vi "Calibration Read Dates.vi"(0 "Equipment Description":T3, 1 "File Path":path=path "C:/GE/Washer DOE/CalibrationDates.txt", 2 "Manufacturer":T3, 3 "Model Number":T3, 5 "error in (no error)":errorcluster, 8 "Calibration ID":T3, 9 "Serial Number":T2, 10 "Last Calibrated":T1 {"Eq20" format="%<%x>T"; "Eq19" format="%<%x>T"; "Eq18" format="%<%x>T"; "Eq17" format="%<%x>T"; "Eq16" format="%<%x>T"; "Eq15" format="%<%x>T"; "Eq14" format="%<%x>T"; "Eq13" format="%<%x>T"; "Eq12" format="%<%x>T"; "Eq11" format="%<%x>T"; "Eq10" format="%<%x>T"; "Eq9" format="%<%x>T"; "Eq8" format="%<%x>T"; "Eq7" format="%<%x>T"; "Eq6" format="%<%x>T"; "Eq5" format="%<%x>T"; "Eq4" format="%<%x>T"; "Eq3" format="%<%x>T"; "Eq2" format="%<%x>T"; "Eq1" format="%<%x>T"}, 11 "Calibration Due":T1 {"Eq20" format="%<%x>T"; "Eq19" format="%<%x>T"; "Eq18" format="%<%x>T"; "Eq17" format="%<%x>T"; "Eq16" format="%<%x>T"; "Eq15" format="%<%x>T"; "Eq14" format="%<%x>T"; "Eq13" format="%<%x>T"; "Eq12" format="%<%x>T"; "Eq11" format="%<%x>T"; "Eq10" format="%<%x>T"; "Eq9" format="%<%x>T"; "Eq8" format="%<%x>T"; "Eq7" format="%<%x>T"; "Eq6" format="%<%x>T"; "Eq5" format="%<%x>T"; "Eq4" format="%<%x>T"; "Eq3" format="%<%x>T"; "Eq2" format="%<%x>T"; "Eq1" format="%<%x>T"}) -> (14 "output cluster":T4 {"Calibration Due"."Eq20" format="%<%x>T"; "Calibration Due"."Eq19" format="%<%x>T"; "Calibration Due"."Eq18" format="%<%x>T"; "Calibration Due"."Eq17" format="%<%x>T"; "Calibration Due"."Eq16" format="%<%x>T"; "Calibration Due"."Eq15" format="%<%x>T"; "Calibration Due"."Eq14" format="%<%x>T"; "Calibration Due"."Eq13" format="%<%x>T"; "Calibration Due"."Eq12" format="%<%x>T"; "Calibration Due"."Eq11" format="%<%x>T"; "Calibration Due"."Eq10" format="%<%x>T"; "Calibration Due"."Eq9" format="%<%x>T"; "Calibration Due"."Eq8" format="%<%x>T"; "Calibration Due"."Eq7" format="%<%x>T"; "Calibration Due"."Eq6" format="%<%x>T"; "Calibration Due"."Eq5" format="%<%x>T"; "Calibration Due"."Eq4" format="%<%x>T"; "Calibration Due"."Eq3" format="%<%x>T"; "Calibration Due"."Eq2" format="%<%x>T"; "Calibration Due"."Eq1" format="%<%x>T"; "Last Calibrated"."Eq20" format="%<%x>T"; "Last Calibrated"."Eq19" format="%<%x>T"; "Last Calibrated"."Eq18" format="%<%x>T"; "Last Calibrated"."Eq17" format="%<%x>T"; "Last Calibrated"."Eq16" format="%<%x>T"; "Last Calibrated"."Eq15" format="%<%x>T"; "Last Calibrated"."Eq14" format="%<%x>T"; "Last Calibrated"."Eq13" format="%<%x>T"; "Last Calibrated"."Eq12" format="%<%x>T"; "Last Calibrated"."Eq11" format="%<%x>T"; "Last Calibrated"."Eq10" format="%<%x>T"; "Last Calibrated"."Eq9" format="%<%x>T"; "Last Calibrated"."Eq8" format="%<%x>T"; "Last Calibrated"."Eq7" format="%<%x>T"; "Last Calibrated"."Eq6" format="%<%x>T"; "Last Calibrated"."Eq5" format="%<%x>T"; "Last Calibrated"."Eq4" format="%<%x>T"; "Last Calibrated"."Eq3" format="%<%x>T"; "Last Calibrated"."Eq2" format="%<%x>T"; "Last Calibrated"."Eq1" format="%<%x>T"}, 19 "error out":errorcluster)   [LabVIEW 2018]
uses:
  Type Definitions/Calibration Time.ctl
  Type Definitions/Calibration.ctl
  Type Definitions/Calibration SN.ctl
  <vilib>/Utility/file.llb/Read Delimited Spreadsheet (string).vi
panel:
  out "file or folder exists?":bool
  in  "Tab Control":enum32{"Controls", "Read Data"}(tab)
  out "Equipment Description":T3
  out "Manufacturer":T3
  out "Model Number":T3
  out "Last Calibrated":T1 {"Eq20" format="%<%x>T"; "Eq19" format="%<%x>T"; "Eq18" format="%<%x>T"; "Eq17" format="%<%x>T"; "Eq16" format="%<%x>T"; "Eq15" format="%<%x>T"; "Eq14" format="%<%x>T"; "Eq13" format="%<%x>T"; "Eq12" format="%<%x>T"; "Eq11" format="%<%x>T"; "Eq10" format="%<%x>T"; "Eq9" format="%<%x>T"; "Eq8" format="%<%x>T"; "Eq7" format="%<%x>T"; "Eq6" format="%<%x>T"; "Eq5" format="%<%x>T"; "Eq4" format="%<%x>T"; "Eq3" format="%<%x>T"; "Eq2" format="%<%x>T"; "Eq1" format="%<%x>T"}
  out "Serial Number":T2
  out "Calibration ID.":T3
  out "Calibration Due":T1 {"Eq20" format="%<%x>T"; "Eq19" format="%<%x>T"; "Eq18" format="%<%x>T"; "Eq17" format="%<%x>T"; "Eq16" format="%<%x>T"; "Eq15" format="%<%x>T"; "Eq14" format="%<%x>T"; "Eq13" format="%<%x>T"; "Eq12" format="%<%x>T"; "Eq11" format="%<%x>T"; "Eq10" format="%<%x>T"; "Eq9" format="%<%x>T"; "Eq8" format="%<%x>T"; "Eq7" format="%<%x>T"; "Eq6" format="%<%x>T"; "Eq5" format="%<%x>T"; "Eq4" format="%<%x>T"; "Eq3" format="%<%x>T"; "Eq2" format="%<%x>T"; "Eq1" format="%<%x>T"}
  out "Size":i32
  out "all rows":string[][](array[string])
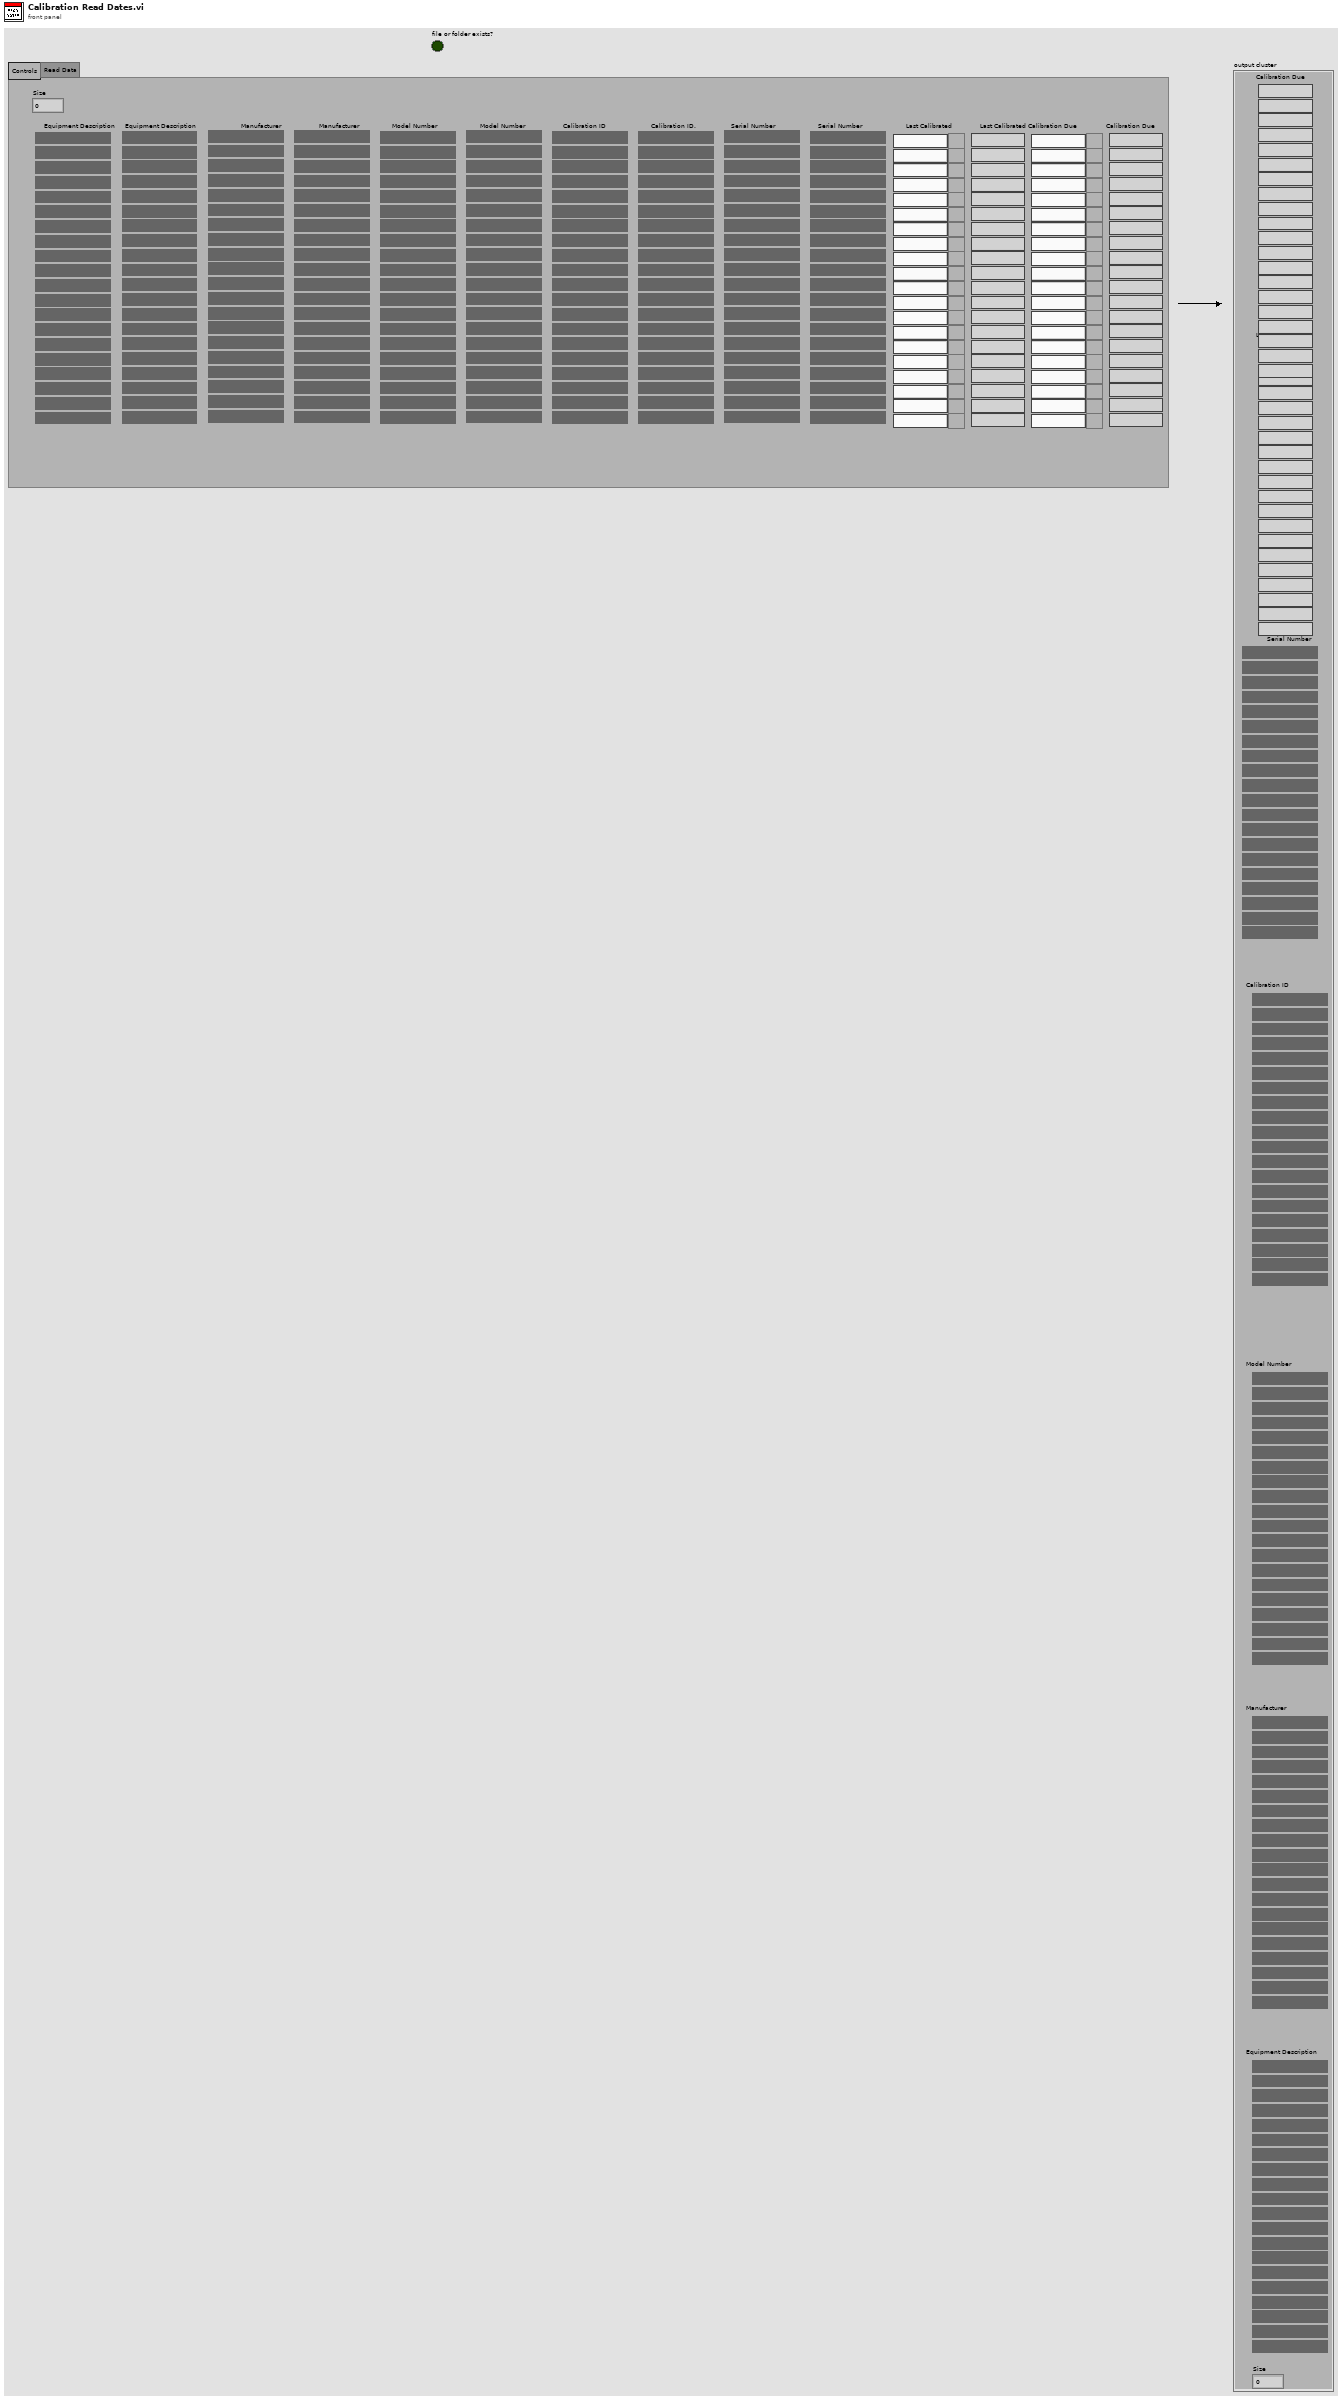
[diagram p1: front panel]
types:
  T1 = typedef "Calibration Time.ctl" = cluster{"Eq1":timestamp, "Eq2":timestamp, "Eq3":timestamp, "Eq4":timestamp, "Eq5":timestamp, "Eq6":timestamp, "Eq7":timestamp, "Eq8":timestamp, "Eq9":timestamp, "Eq10":timestamp, "Eq11":timestamp, "Eq12":timestamp, "Eq13":timestamp, "Eq14":timestamp, "Eq15":timestamp, "Eq16":timestamp, "Eq17":timestamp, "Eq18":timestamp, "Eq19":timestamp, "Eq20":timestamp}
  T2 = typedef "Calibration SN.ctl" = cluster{"Eq 1":string, "Eq 2":string, "Eq 3":string, "Eq 4":string, "Eq 5":string, "Eq 6":string, "Eq 7":string, "Eq 8":string, "Eq 9":string, "Eq 10":string, "Eq 11":string, "Eq 12":string, "Eq 13":string, "Eq 14":string, "Eq 15":string, "Eq 16":string, "Eq 17":string, "Eq 18":string, "Eq 19":string, "Eq 20":string}
  T3 = typedef "Calibration.ctl" = cluster{"Eq 1":string, "Eq 2":string, "Eq 3":string, "Eq 4":string, "Eq 5":string, "Eq 6":string, "Eq 7":string, "Eq 8":string, "Eq 9":string, "Eq 10":string, "Eq 11":string, "Eq 12":string, "Eq 13":string, "Eq 14":string, "Eq 15":string, "Eq 16":string, "Eq 17":string, "Eq 18":string, "Eq 19":string, "Eq 20":string}
  T4 = cluster{"Calibration Due":T1, "Last Calibrated":T1, "Serial Number":T2, "Calibration ID":T3, "Model Number":T3, "Manufacturer":T3, "Equipment Description":T3, "Size":i32}
  T5 = enum16{"open", "replace", "create", "open or create", "replace or create", "replace or create with confirmation"}
  T6 = cluster{"Calibration Due out":T1, "Calibration Due out":T1, "Serial Number out":T2, "Serial Number out":T2, "Serial Number out":T2, "Serial Number out":T2, "Serial Number out":T2, "size(s)":i32}
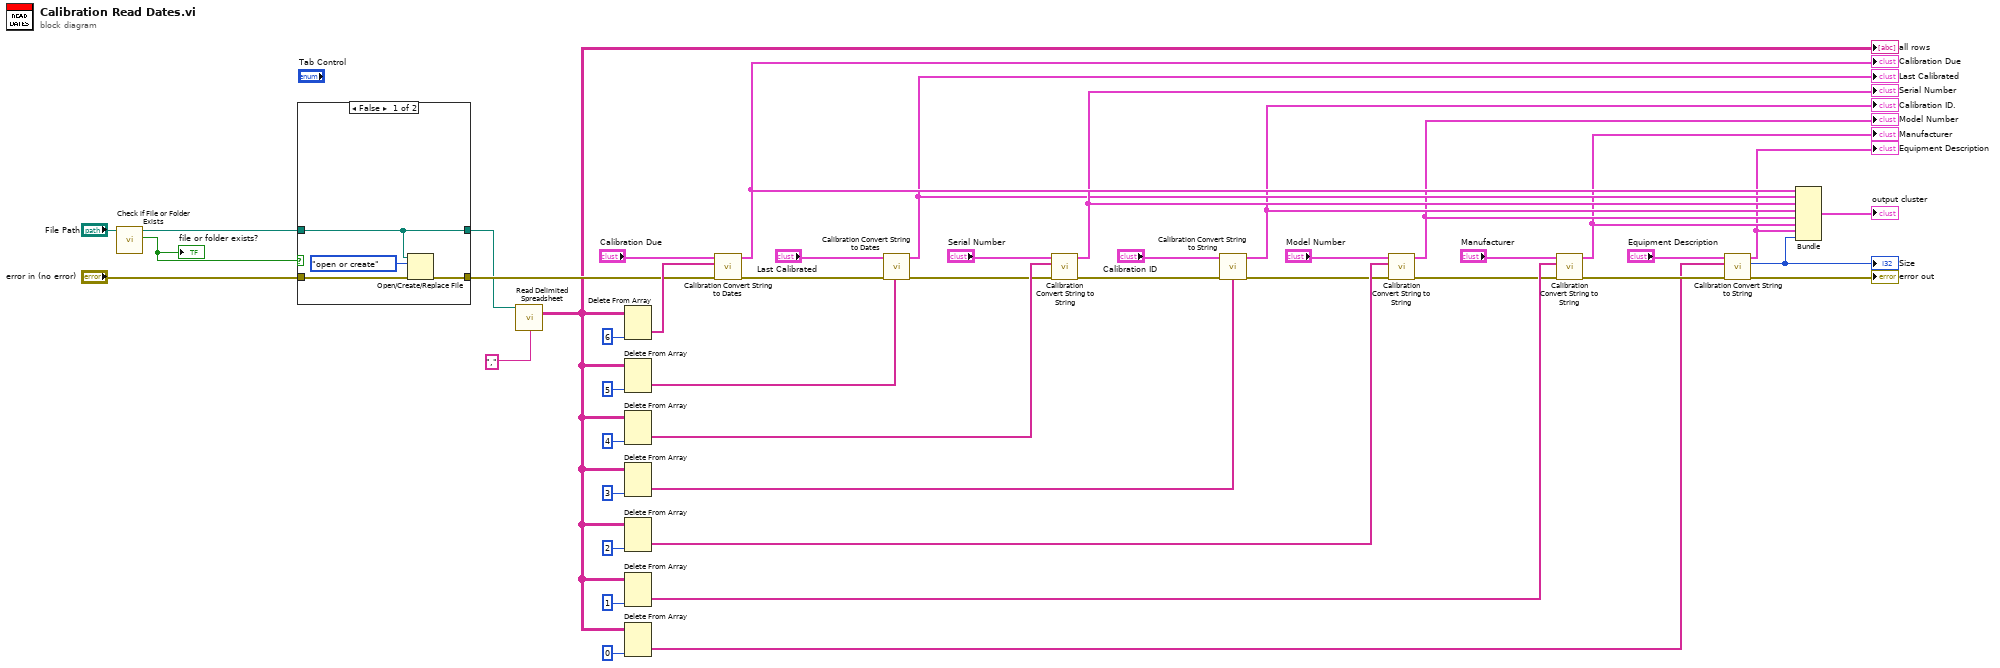
[diagram p0: block diagram]
diagram:
  n1 = call <vilib>:"Check if File or Folder Exists.vi"("path"="File Path") -> ("file or folder exists?"=w29:bool, "dup path"=w28:path)  [unwired: 8 in, 1 out]
  "file or folder exists?" <- w29
  n2 = case shown="False" w29 {
    tunnel: w28 -> [w46 w50]
    tunnel: "error in (no error)" -> [w48 w51]
    tunnel: [w47 w51] -> w26
    tunnel: [w46 w50] -> w25
    frame False {
      n3 = Open/Create/Replace File(file path (use dialog)=w46, error in=w48, operation (0:open)=T5."open or create") -> (error out=w47:errorcluster)  [unwired: 3 in, 2 out]
    }
    frame True {
    }
  }
  n4 = call-poly <vilib>:"Read Delimited Spreadsheet.vi"("file path (dialog if empty)"=w25, "delimiter (\\t)"="," ("delimiter (\\t)")) -> ("all rows"=w1:string[][])  [unwired: 8 in, 5 out]
  "all rows" <- w1
  n5 = Delete From Array(array=w1, index (col)=6 ("disabled index (col)")) -> (deleted portion=w40:string[])  [unwired: 2 in, 1 out]
  n6 = Delete From Array(array=w1, index (col)=5 ("disabled index (col)")) -> (deleted portion=w24:string[])  [unwired: 2 in, 1 out]
  n7 = Delete From Array(array=w1, index (col)=4 ("disabled index (col)")) -> (deleted portion=w36:string[])  [unwired: 2 in, 1 out]
  n8 = Delete From Array(array=w1, index (col)=3 ("disabled index (col)")) -> (deleted portion=w18:string[])  [unwired: 2 in, 1 out]
  n9 = Delete From Array(array=w1, index (col)=2 ("disabled index (col)")) -> (deleted portion=w15:string[])  [unwired: 2 in, 1 out]
  n10 = Delete From Array(array=w1, index (col)=1 ("disabled index (col)")) -> (deleted portion=w11:string[])  [unwired: 2 in, 1 out]
  n11 = Delete From Array(array=w1, index (col)=0 ("disabled index (col)")) -> (deleted portion=w3:string[])  [unwired: 2 in, 1 out]
  n12 = call "Calibration Convert String to Dates.vi"("error in (no error)"=w26, "all rows"=w40, "Calibration Due in"="Calibration Due") -> ("error out"=w22:errorcluster, "Calibration Due out"=w33:T1)  [unwired: 7 in]
  "Calibration Due" <- w33
  n13 = call "Calibration Convert String to Dates.vi"("error in (no error)"=w22, "all rows"=w24, "Calibration Due in"="Last Calibrated") -> ("error out"=w20:errorcluster, "Calibration Due out"=w21:T1)  [unwired: 7 in]
  "Last Calibrated" <- w21
  n14 = call "Calibration Convert String to String.vi"("error in (no error)"=w20, "all rows"=w36, "Serial Number in"="Serial Number") -> ("error out"=w17:errorcluster, "Serial Number out"=w32:T2)  [unwired: 6 in, 1 out]
  "Serial Number" <- w32
  n15 = call "Calibration Convert String to String.vi"("error in (no error)"=w17, "all rows"=w18, "Serial Number in"="Calibration ID") -> ("error out"=w13:errorcluster, "Serial Number out"=w16:T2)  [unwired: 6 in, 1 out]
  "Calibration ID." <- w16
  n16 = call "Calibration Convert String to String.vi"("error in (no error)"=w13, "all rows"=w15, "Serial Number in"="Model Number") -> ("error out"=w9:errorcluster, "Serial Number out"=w12:T2)  [unwired: 6 in, 1 out]
  "Model Number" <- w12
  n17 = call "Calibration Convert String to String.vi"("error in (no error)"=w9, "all rows"=w11, "Serial Number in"="Manufacturer") -> ("error out"=w6:errorcluster, "Serial Number out"=w8:T2)  [unwired: 6 in, 1 out]
  "Manufacturer" <- w8
  n18 = call "Calibration Convert String to String.vi"("error in (no error)"=w6, "all rows"=w3, "Serial Number in"="Equipment Description") -> ("error out"=→"error out":errorcluster, "size(s)"=w2:i32, "Serial Number out"=w5:T2)  [unwired: 6 in]
  "Size" <- w2
  "Equipment Description" <- w5
  n19 = Bundle("Calibration Due out"=w33, "Calibration Due out"=w21, "Serial Number out"=w32, "Serial Number out"=w16, "Serial Number out"=w12, "Serial Number out"=w8, "Serial Number out"=w5, "size(s)"=w2) -> (→"output cluster":T6)  [unwired: 1 in]
